vi "Error_Clear.vi"(8 "error in":errorcluster) -> (0 "error out (no error)":errorcluster)   [LabVIEW 2020, in "hse-misc.lvlib"]
doc: "Clears the error in <b>error in</b>\n\n\n\n____\nHAMPEL SOFTWARE ENGINEERING v3.8.0 (2023-12-18 14:41)"
uses:
  hse-misc.lvlib
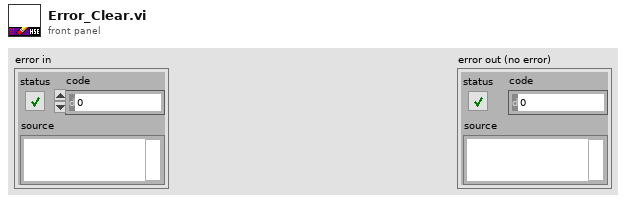
[diagram p1: front panel]
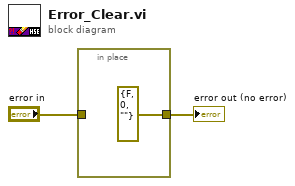
[diagram p0: block diagram]
diagram:
  n1 = in-place {
    in-place-border: [errorcluster {"status"=FALSE, "code"=0, "source"=""} ("error out")] -> w2
    in-place-border: "error in" -> [_]
  }
  "error out (no error)" <- w2
